vi "ASCReadBaseTime.vi"(10 "偏置时间":string, 11 "ASC首行":string) -> (3 "基时间簇":T1)   [LabVIEW 2015]
uses:
  <vilib>/Utility/miscctls.llb/LVDateTimeRec.ctl
  <vilib>/regexp/Match Regular Expression.xnode
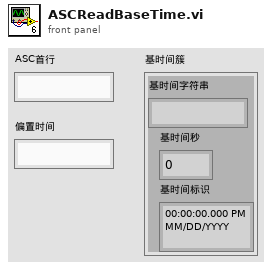
[diagram p1: front panel]
types:
  T1 = cluster{"基时间字符串":string, "基时间秒":dbl, "基时间标识":timestamp}
  T2 = typedef "LVDateTimeRec.ctl" = cluster{"fractional second":dbl, "second":i32, "minute":i32, "hour":i32, "day of month":i32, "month":i32, "year":i32, "day of week":i32, "day of year":i32, "DST":i32}
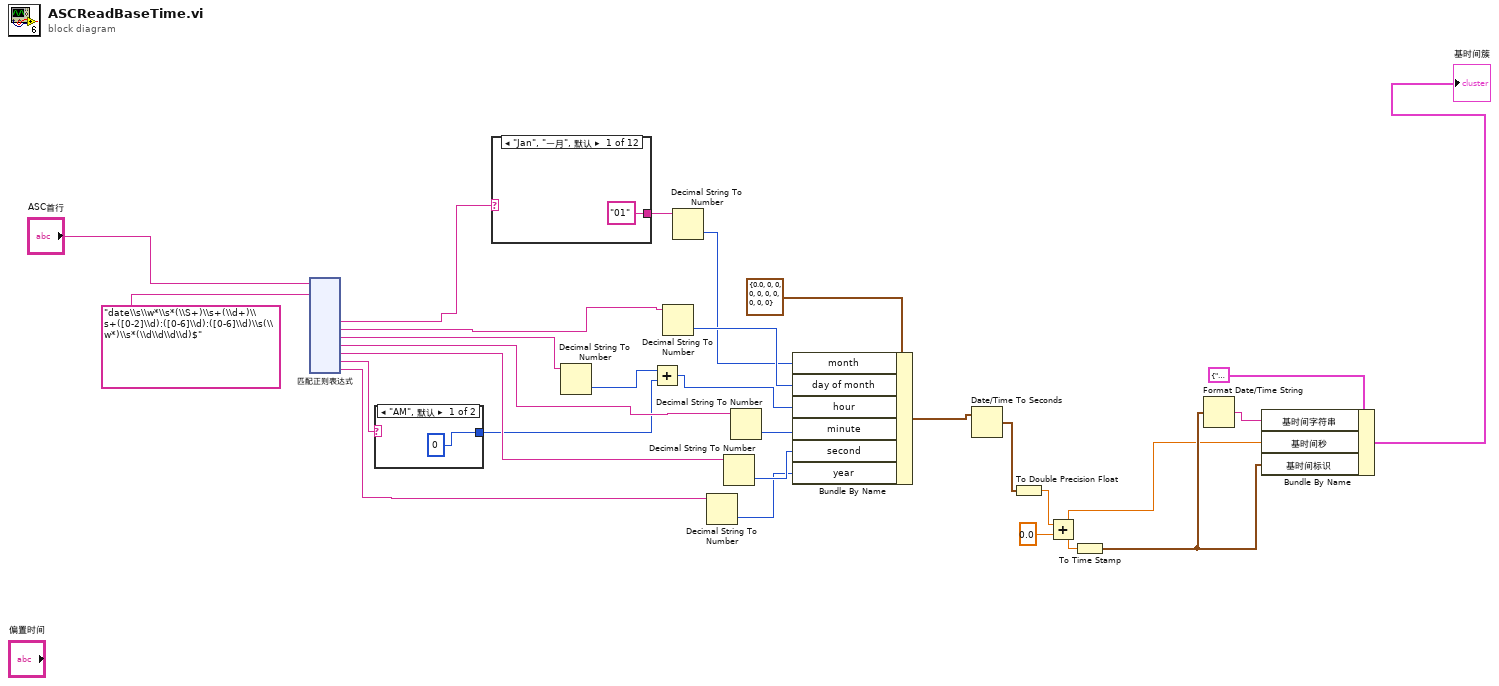
[diagram p0: block diagram]
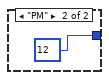
[diagram p2: hidden frame]
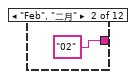
[diagram p3: hidden frame]
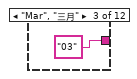
[diagram p4: hidden frame]
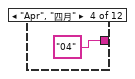
[diagram p5: hidden frame]
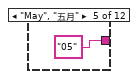
[diagram p6: hidden frame]
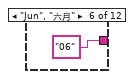
[diagram p7: hidden frame]
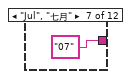
[diagram p8: hidden frame]
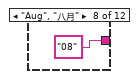
[diagram p9: hidden frame]
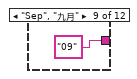
[diagram p10: hidden frame]
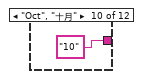
[diagram p11: hidden frame]
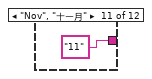
[diagram p12: hidden frame]
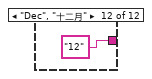
[diagram p13: hidden frame]
diagram:
  n1 = xnode "匹配正则表达式"("输入字符串"="ASC首行", "正则表达式"="date\\s\\w*\\s*(\\S+)\\s+(\\d+)\\s+([0-2]\\d):([0-6]\\d):([0-6]\\d)\\s(\\w*)\\s*(\\d\\d\\d\\d)$") -> ("子匹配 1"=w9:string, "子匹配 2"=w19:string, "子匹配 3"=w18:string, "子匹配 4"=w17:string, "子匹配 5"=w15:string, "子匹配 6"=w3:string, "子匹配 7"=w6:string)  [unwired: 4 in, 5 out]
  n2 = case shown="\"AM\", 默认" w3 {
    tunnel: [0 12] -> w2
    frame "AM", Default {
    }
    frame "PM" {
    }
  }
  n3 = case shown="\"Jan\", \"一月\", 默认" w9 {
    tunnel: ["01" "02" "03" "04" "05" "06" "07" "08" "09" "10" "11" "12"] -> w11
    frame "Jan", "一月", Default {
    }
    frame "Feb", "二月" {
    }
    frame "Mar", "三月" {
    }
    frame "Apr", "四月" {
    }
    frame "May", "五月" {
    }
    frame "Jun", "六月" {
    }
    frame "Jul", "七月" {
    }
    frame "Aug", "八月" {
    }
    frame "Sep", "九月" {
    }
    frame "Oct", "十月" {
    }
    frame "Nov", "十一月" {
    }
    frame "Dec", "十二月" {
    }
  }
  n4 = Decimal String To Number(string=w18) -> (number=w5:i32)  [unwired: 2 in, 1 out]
  n5 = Add(x=w5, y=w2) -> (x+y=w4:i32)
  n6 = Decimal String To Number(string=w19) -> (number=w20:i32)  [unwired: 2 in, 1 out]
  n7 = Decimal String To Number(string=w11) -> (number=w12:i32)  [unwired: 2 in, 1 out]
  n8 = Decimal String To Number(string=w6) -> (number=w13:i32)  [unwired: 2 in, 1 out]
  n9 = Decimal String To Number(string=w15) -> (number=w14:i32)  [unwired: 2 in, 1 out]
  n10 = Decimal String To Number(string=w17) -> (number=w16:i32)  [unwired: 2 in, 1 out]
  n11 = Bundle By Name(cluster=T2 {"fractional second"=0.0, "second"=0, "minute"=0, "hour"=0, "day of month"=0, "month"=0, "year"=0, "day of week"=0, "day of year"=0, "DST"=0} ("日期时间记录"), "month"=w12, "day of month"=w20, "hour"=w4, "minute"=w16, "second"=w14, "year"=w13) -> (w21:T2)
  n12 = Date/Time To Seconds(2:w21) -> (0:w22:timestamp)  [unwired: 1 in]
  n13 = To Double Precision Float(number=w22) -> (double precision float=w23:dbl)
  n14 = Add(x=w23, y=0.0) -> (x+y=w25:dbl)
  n15 = To Time Stamp(1:w25) -> (0:w26:timestamp)
  n16 = Format Date/Time String(seconds (now)=w26) -> (date/time string=w27:string)  [unwired: 2 in]
  n17 = Bundle By Name(cluster=T1 {"基时间字符串"="1904/1/1 8:00:00", "基时间秒"=0.0, "基时间标识"=timestamp(0 s since 1904-01-01)} ("基时间簇"), "基时间字符串"=w27, "基时间秒"=w25, "基时间标识"=w26) -> (→"基时间簇":T1)
